vi "Tosca-Check For Track Switch.vi"(0 "Finished in":bool, 2 "Analysis In":T1, 5 "reversal":bool, 9 "which in":i32, 11 "nacq":i32, 12 "Switch after":i32, 13 "Switch type":enum16{"Trials", "Reversals"}(ring)) -> (4 "Finished out":bool, 10 "which out":i32, 15 "nacq out":i32)   [LabVIEW 2020]
uses:
  Typedefs/Tosca-Analysis State.ctl
  Typedefs/Tosca-Adaptation State.ctl
  Typedefs/Tosca-Adaptation Track State.ctl
  Typedefs/Tosca-Adaptation History Element.ctl
  Classes/Parameters/Histogram Data.ctl
  Classes/Parameters/Connect.ctl
  Classes/Parameters/Parameters.lvclass
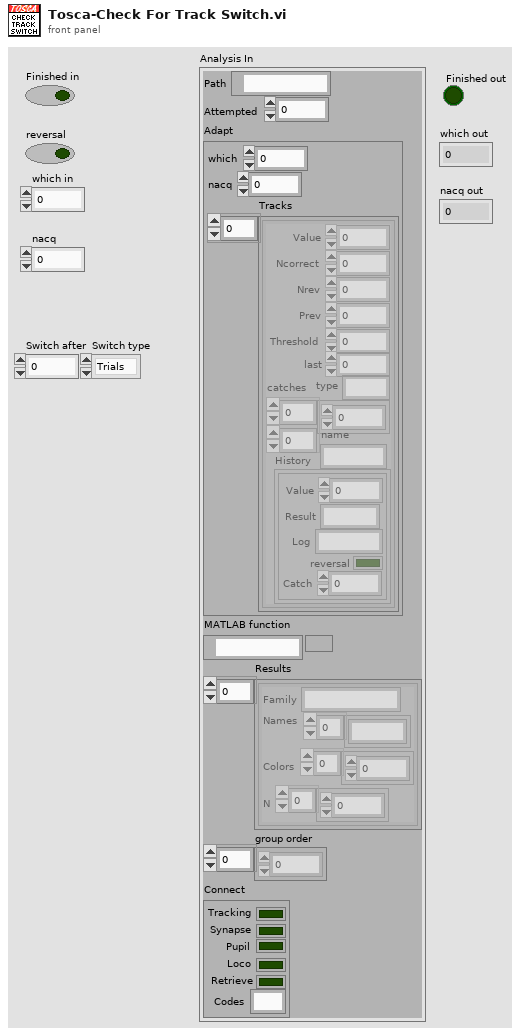
[diagram p1: front panel]
types:
  T1 = typedef "Tosca-Analysis State.ctl" = cluster{"Path":path, "Attempted":i32, "Adapt":T2, "MATLAB function":path, "Results":T5[], "group order":i32[], "Connect":T6}
  T2 = typedef "Tosca-Adaptation State.ctl" = cluster{"which":i32, "nacq":i32, "Tracks":T3[]}
  T3 = typedef "Tosca-Adaptation Track State.ctl" = cluster{"Value":dbl, "Ncorrect":i32, "Nrev":i32, "Prev":dbl, "History":T4[], "Threshold":dbl, "last":i32, "type":string, "catches":dbl[][], "name":string}
  T4 = typedef "Tosca-Adaptation History Element.ctl" = cluster{"Value":dbl, "Result":string, "Log":string, "reversal":bool, "Catch":dbl}
  T5 = typedef "Parameters.lvclass/Histogram Data.ctl" = cluster{"Family":string, "Names":string[], "Colors":u32[], "N":i32[]}
  T6 = typedef "Parameters.lvclass/Connect.ctl" = cluster{"Tracking":bool, "Synapse":bool, "Pupil":bool, "Loco":bool, "Retrieve":bool, "Codes":string}
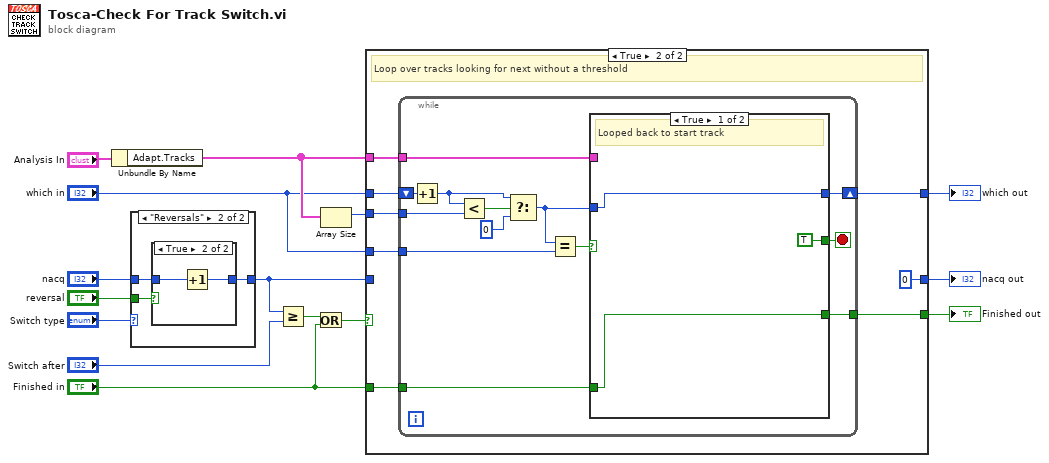
[diagram p0: block diagram]
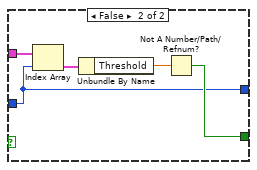
[diagram p3: hidden frame]
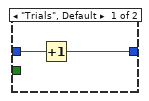
[diagram p4: hidden frame]
diagram:
  n1 = Unbundle By Name("Analysis In") -> ("Adapt.Tracks"=w5:T3[])
  n2 = case shown="\"Reversals\"" "Switch type" {
    tunnel: "nacq" -> [w17 w19]
    tunnel: [w16 w18] -> w9
    tunnel: "reversal" -> [_ w20]
    frame "Trials", Default {
      n3 = Increment(x=w17) -> (x+1=w16:i32)
    }
    frame "Reversals" {
      n4 = case shown="True" w20 {
        tunnel: w19 -> [w21 w23]
        tunnel: [w21 w22] -> w18
        frame False {
        }
        frame True {
          n5 = Increment(x=w23) -> (x+1=w22:i32)
        }
      }
    }
  }
  n6 = Greater Or Equal?(x=w9, y="Switch after") -> (x >= y?=w11:bool)
  n7 = Or(x=w11, y="Finished in") -> (x .or. y?=w10:bool)
  n8 = Array Size(array=w5) -> (size(s)=w6:i32)
  n9 = case shown="True" w10 {
    tunnel: "which in" -> [w24 w28]
    tunnel: w9 -> [w25 _]
    tunnel: [w25 0 ("nacq")] -> w8
    tunnel: w5 -> [_ w33]
    tunnel: w6 -> [_ w32]
    tunnel: "which in" -> [_ w31]
    tunnel: [_ w30] -> w3
    tunnel: [w24 w29] -> w2
    tunnel: "Finished in" -> [_ w26]
    frame False {
    }
    frame True {
      # "Loop over tracks looking for next without a threshold"
      n10 = while {
        shift-right: [w36] -> w29
        shift-left: w28 -> [w44]
        tunnel: w33 -> [w39]
        tunnel: w32 -> [w45]
        tunnel: w31 -> [w42]
        tunnel: [w37] -> w30
        tunnel: w26 -> [w34]
        stop <- w38 stop-if-true
        n11 = Increment(x=w44) -> (x+1=w35:i32)
        n12 = Less?(x=w35, y=w45) -> (x < y?=w46:bool)
        n13 = Select(t=w35, s=w46, f=0) -> (s? t:f=w40:i32)
        n14 = Equal?(x=w40, y=w42) -> (x = y?=w41:bool)
        n15 = case shown="True" w41 {
          tunnel: w40 -> [w49 w50]
          tunnel: w39 -> [_ w54]
          tunnel: [TRUE w51] -> w38
          tunnel: [w47 _] -> w37
          tunnel: [w49 w50] -> w36
          tunnel: w34 -> [w47 _]
          frame True {
            # "Looped back to start track"
          }
          frame False {
            n16 = Index Array(array=w54, index=w50) -> (element=w53:T3)
            n17 = Unbundle By Name(w53) -> ("Threshold"=w52:dbl)
            n18 = Not A Number/Path/Refnum?(number/path/refnum=w52) -> (NaN/Path/Refnum?=w51:bool)
          }
        }
      }
    }
  }
  "Finished out" <- w3
  "nacq out" <- w8
  "which out" <- w2
